vi "ConfigureMemory.vi"(8 "Error In":errorcluster, 10 "Channel Patterns":string[](array[string]), 11 "Keithley 7001 In":refnum<visa-resource-name>) -> (0 "Error Out":errorcluster, 3 "Keithley 7001 Out":refnum<visa-resource-name>)   [LabVIEW 2012]
uses:
  driver/Public/Controls/Slot.ctl
  driver/Keithley-7001.lvlib
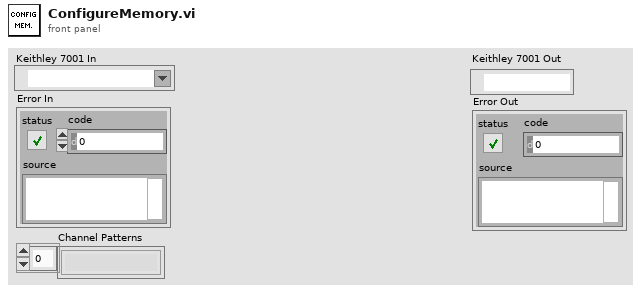
[diagram p1: front panel]
types:
  T1 = typedef "Keithley-7001.lvlib/Slot.ctl" = enum16{"Slot 1", "Slot 2"}
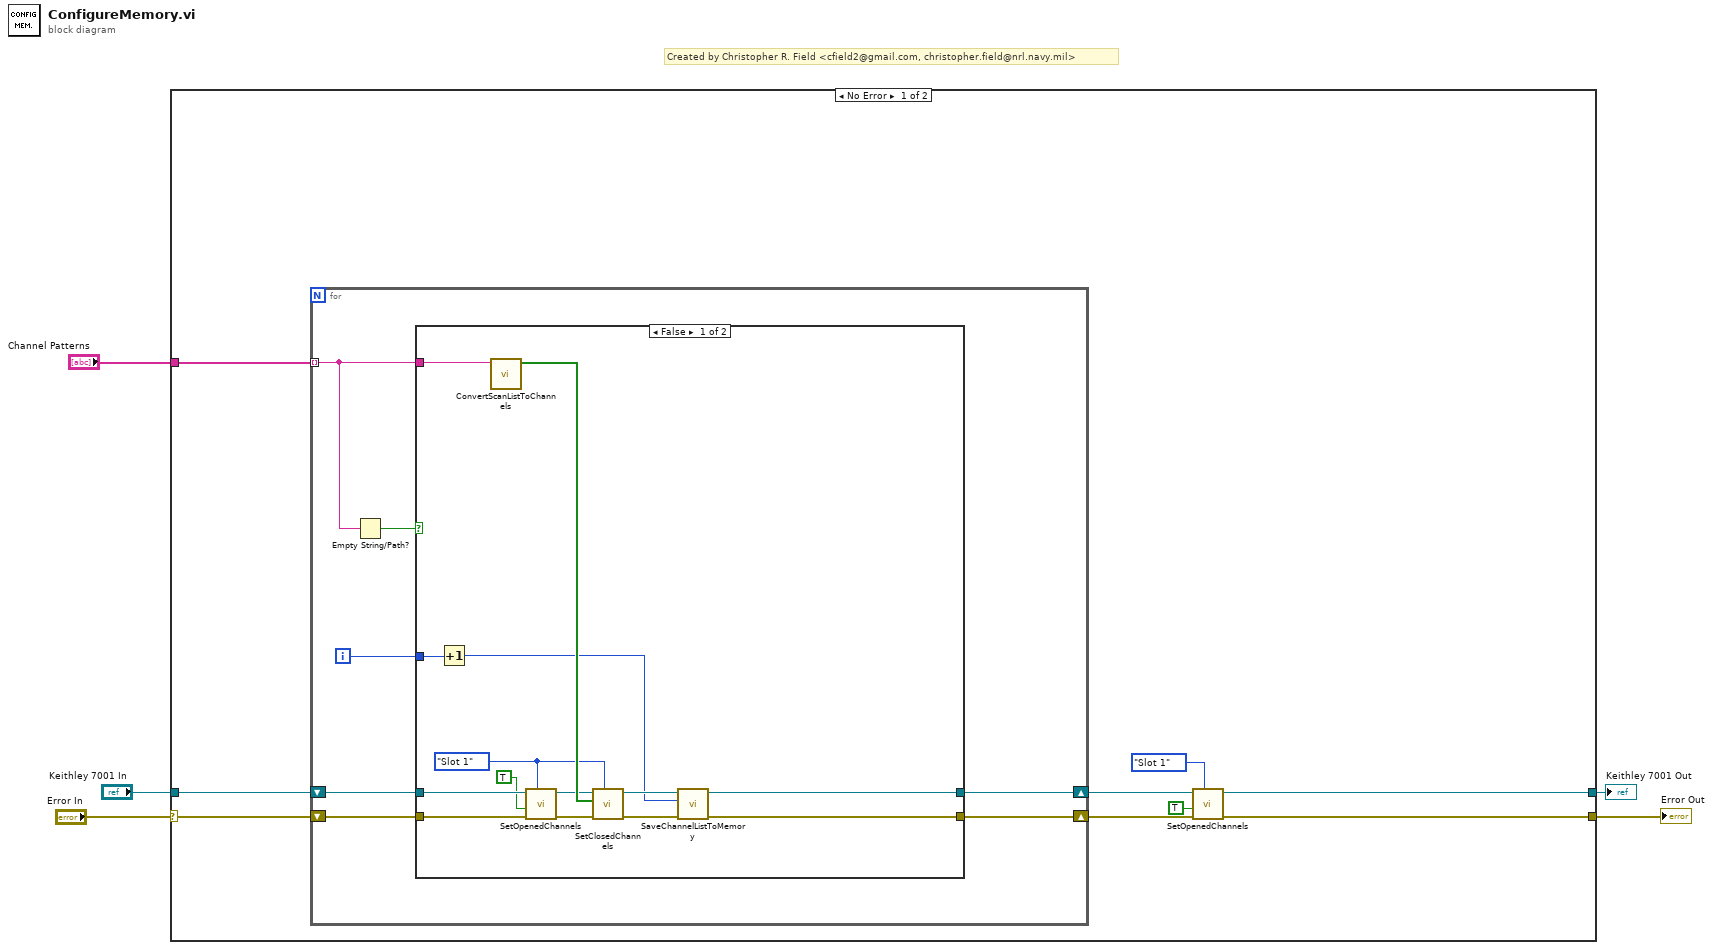
[diagram p0: block diagram]
diagram:
  # "Created by Christopher R. Field <cfield2@gmail.com, christopher.field@nrl.navy.mil>"
  n1 = case shown="No Error" "Error In" {
    selector: "Error In" -> [w13 w38]
    tunnel: "Keithley 7001 In" -> [w14 w39]
    tunnel: [w8 w39] -> w3
    tunnel: [w7 w38] -> w2
    tunnel: "Channel Patterns" -> [w6 _]
    frame No Error {
      n2 = for {
        tunnel: w6 -> [w17] mode=indexing
        shift-right: [w18] -> w12
        shift-left: w14 -> [w21]
        shift-right: [w19] -> w11
        shift-left: w13 -> [w20]
        i -> [w15]
        n3 = Empty String/Path?(string/path=w17) -> (empty?=w16:bool)
        n4 = case shown="False" w16 {
          tunnel: w21 -> [w34 w37]
          tunnel: w20 -> [w30 w36]
          tunnel: [w26 w36] -> w19
          tunnel: [w25 w37] -> w18
          tunnel: w17 -> [w24 _]
          tunnel: w15 -> [w23 _]
          frame False {
            w33 = Slot."Slot 1" ("Slot")
            n5 = Increment(x=w23) -> (x+1=w22:i32)
            n6 = call "ConvertScanListToChannels.vi"("Scan List"=w24) -> ("Channels"=w35:bool[])  [unwired: 10 in]
            n7 = call "SetOpenedChannels.vi"("Slot"=w33, "Error In"=w30, "All?"=TRUE, "Keithley 7001 In"=w34) -> ("Error Out"=w31:errorcluster, "Keithley 7001 Out"=w32:refnum<visa-resource-name>)  [unwired: 6 in]
            n8 = call "SetClosedChannels.vi"("Slot"=w33, "Error In"=w31, "Channels"=w35, "Keithley 7001 In"=w32) -> ("Error Out"=w27:errorcluster, "Keithley 7001 Out"=w28:refnum<visa-resource-name>)  [unwired: 6 in]
            n9 = call "SaveChannelListToMemory.vi"("Error In"=w27, "Memory Location (1-100)"=w22, "Keithley 7001 In"=w28) -> ("Error Out"=w26:errorcluster, "Keithley 7001 Out"=w25:refnum<visa-resource-name>)  [unwired: 7 in]
          }
          frame True {
          }
        }
      }
      n10 = call "SetOpenedChannels.vi"("Slot"=Slot."Slot 1", "Error In"=w11, "All?"=TRUE, "Keithley 7001 In"=w12) -> ("Error Out"=w7:errorcluster, "Keithley 7001 Out"=w8:refnum<visa-resource-name>)  [unwired: 6 in]
    }
    frame Error {
    }
  }
  "Keithley 7001 Out" <- w3
  "Error Out" <- w2
